vi "Calculate Color Index Array.vi"(8 "error in (no error)":errorcluster, 10 "3D Plot Datatype in":refnum<class "3D Plot Datatype.lvclass">, 11 "Plot Representation In":T1) -> (0 "error out":errorcluster, 2 "3D Plot Datatype out":refnum<class "3D Plot Datatype.lvclass">, 3 "Plot Representation Out":T1)   [LabVIEW 2020, in "3D Plot Datatype.lvclass"]
uses:
  3D Plot Datatype.lvclass
  Plot Representation.ctl
  Range Clusters.ctl
  Mesh Data.ctl
  3D Plot.lvclass
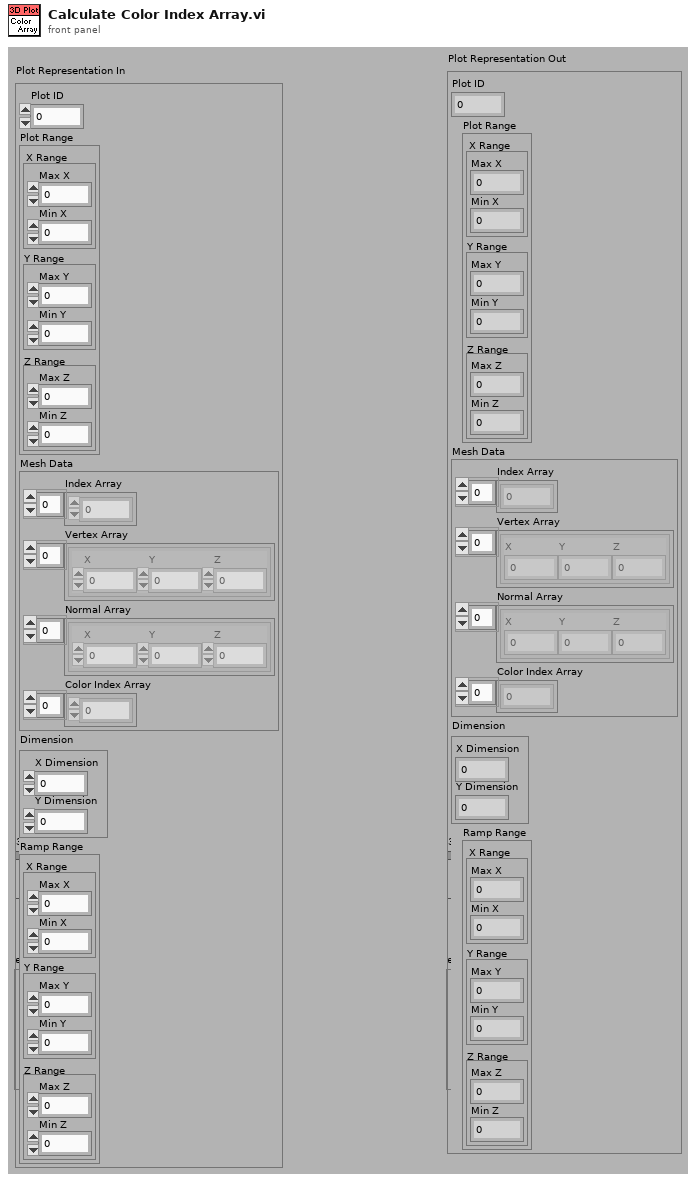
[diagram p1: front panel]
types:
  T1 = typedef "3D Plot.lvclass/Plot Representation.ctl" = cluster{"Plot ID":i32, "Plot Range":T2, "Mesh Data":T3, "Dimension":cluster{"X Dimension":i32, "Y Dimension":i32}, "Ramp Range":T2}
  T2 = typedef "3D Plot.lvclass/Range Clusters.ctl" = cluster{"X Range":cluster{"Max X":sgl, "Min X":sgl}, "Y Range":cluster{"Max Y":sgl, "Min Y":sgl}, "Z Range":cluster{"Max Z":sgl, "Min Z":sgl}}
  T3 = typedef "3D Plot.lvclass/Mesh Data.ctl" = cluster{"Index Array":u32[], "Vertex Array":cluster{"X":sgl, "Y":sgl, "Z":sgl}[], "Normal Array":cluster{"X":sgl, "Y":sgl, "Z":sgl}[], "Color Index Array":i32[]}
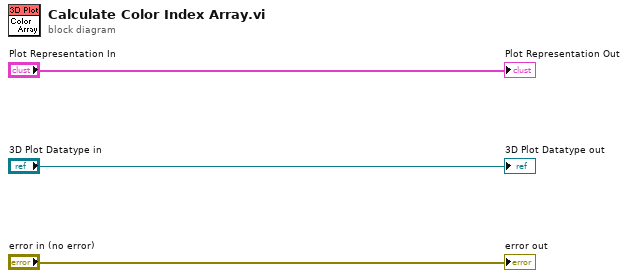
[diagram p0: block diagram]
diagram:
  "error out" <- "error in (no error)"
  "3D Plot Datatype out" <- "3D Plot Datatype in"
  "Plot Representation Out" <- "Plot Representation In"
